vi "HVPSS_Single.vi"(0 "address":string="10.47.1.10", 1 "remote port or service name":u16=7, 4 "CONNECT":bool, 5 "SET":bool, 7 "FIFO_SIZE":u32=100, 9 "TRIG_DELAY":u32=50, 11 "TRIGGER_LEVEL":u32=10) -> (14 "Oscilloscope":waveform(dbl)(graph), 15 "DATA_AVAILABLE":bool, 18 "Timestamp":u64 format="%.0x", 19 "Halt":bool)   [LabVIEW 2019]
uses:
  Histogram/Histogram.lvlib
  <vilib>/Analysis/NI_AAL_SigProc.lvlib
  <vilib>/Analysis/NI_AALBase.lvlib
panel:
  in  "Tab Control":enum32{"ADC and Decimator", "pAmp CTRL"}(tab)
  in  "Full Scale Range":bool
  in  "DDR":bool
  in  "DCLK_RST":bool
  in  "ON":bool=TRUE
  in  "LED 1":bool
  in  "LED 0":bool=TRUE
  in  "CAL":bool
  in  "CAL_DLY":bool
  in  "OUTV":bool
  out "ADC500_CFG":u32=128
  in  "N":u32=1
  out "number":u32=9
  in  "SET POTS":bool
  in  "FINE OFFSET":u16(slide)=1023 scale=0.0..1023.0
  in  "OFFSET":u16(slide)=1023 scale=0.0..1024.0
  in  "HV_CTRL":bool
  out "RANGE 2":bool=TRUE
  out "RANGE 1":bool
  in  "RANGE":bool
  in  "LED":bool=TRUE
  in  "INIT":bool
  in  "Tab Control 2":T1(tab)
  in  "Trigger Edge":u32(ring)=3 items=["Falling Edge", "Rising Edge", "Auto", "EXT"]
  in  "CONTINOUS":bool
  in  "Counts":u32
  in  "GEN HISTO":bool
  in  "ENABLE":bool
  out "HISTOGRAM":u32[](graph)
  out "DONE":bool
  out "Progress":u32(slide) max=0
  out "STATUS":u32
  in  "Store Data":bool
  out "pAs_STATUS":u8[](array[numeric])=[1, 0, 0, 0, 9, 0, 0, 0]
  out "PAM_INIT_STATUS":u8[](array[numeric])
  out "ADC500_STATUS":u8[](array[numeric])
  out "DEC_STATUS":u8[](array[numeric])
  out "CONNECTED":bool
  out "BUSY":bool
  in  "Filename":path=path "/media/kbo/DATA/cernbox/DATA20211012/Cs137_dec2/Cs137_dec2.xlsx"
  out "output waveform":waveform(dbl)
  in  "threshold":dbl format="%0.2f"
  in  "width":i32=3 min=3
  in  "initialize (T)":bool=TRUE
  out "# found":i32
  out "Amplitudes":dbl[](array[numeric])
  in  "# bins":i32
  out "Histogram Graph":T2(graph)
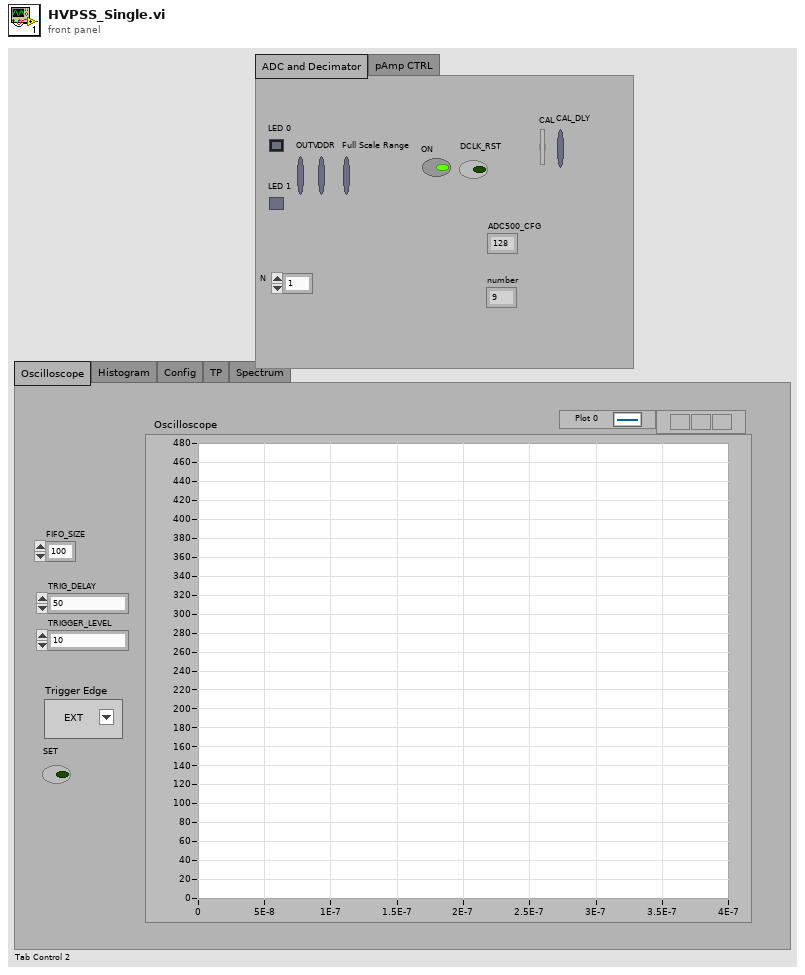
[diagram p1: front panel]
types:
  T1 = enum32{"Oscilloscope", "Histogram", "Config", "TP", "Spectrum"}
  T2 = cluster{"X Values":dbl[], "Histogram: h(x)":i32[]}
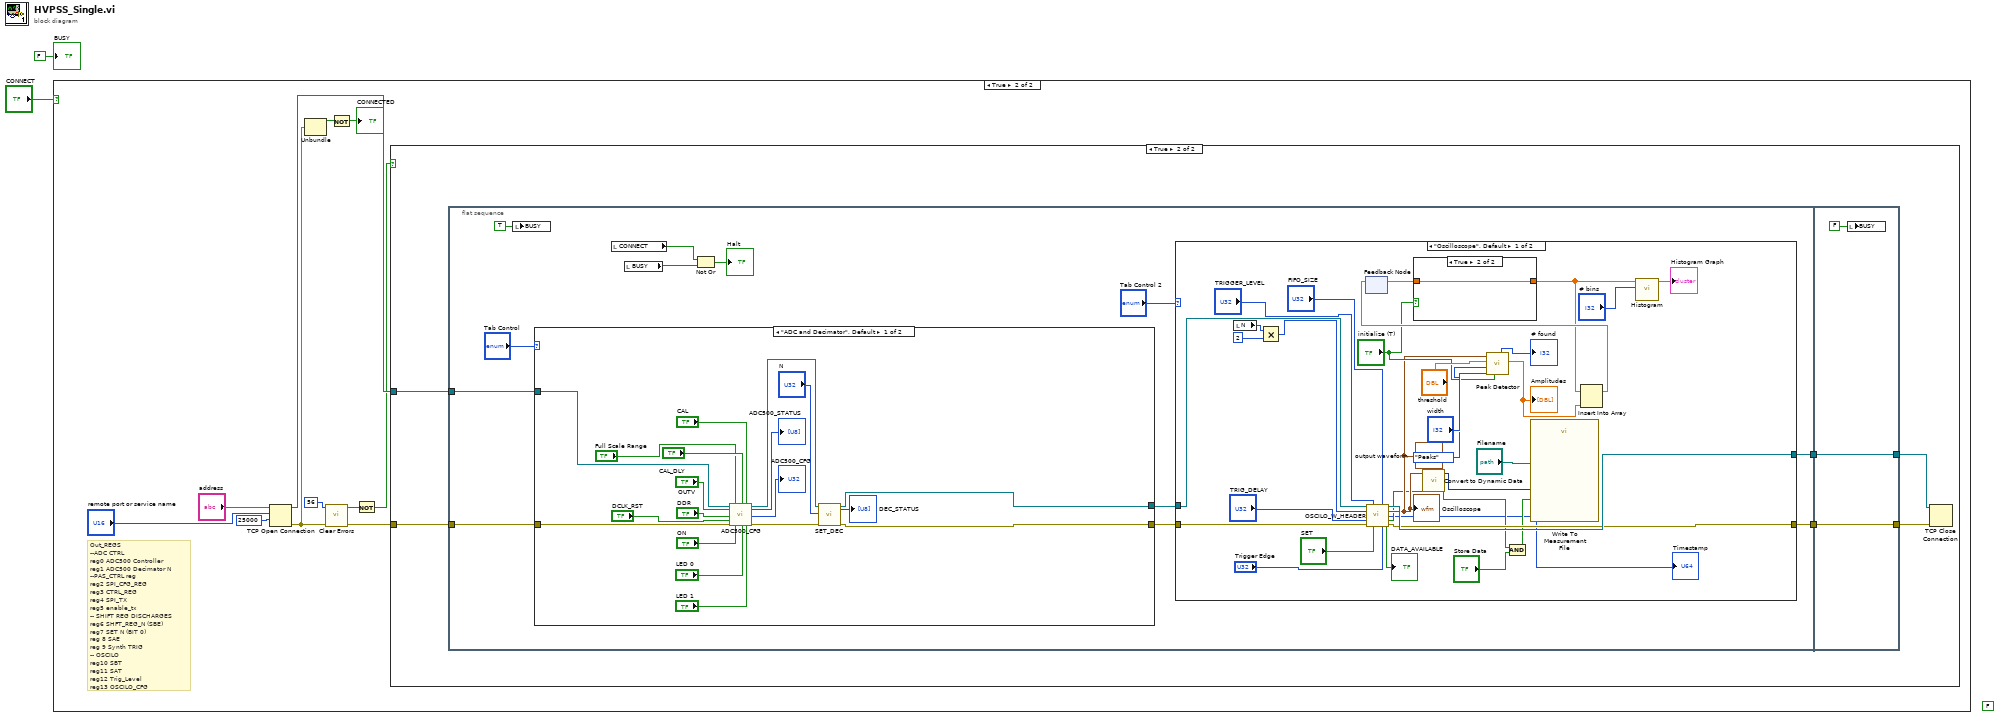
[diagram p0: block diagram]
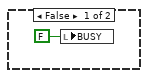
[diagram p3: hidden frame]
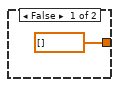
[diagram p4: hidden frame]
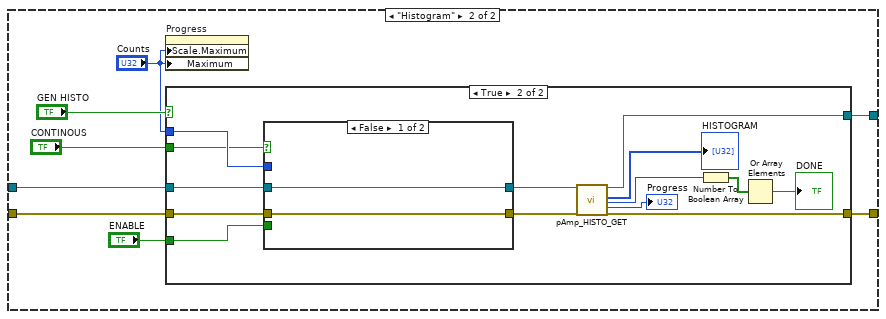
[diagram p5: hidden frame]
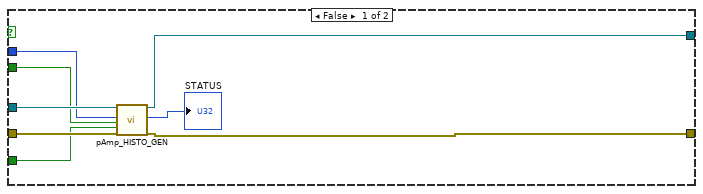
[diagram p6: hidden frame]
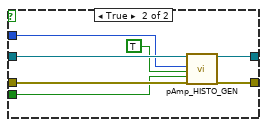
[diagram p7: hidden frame]
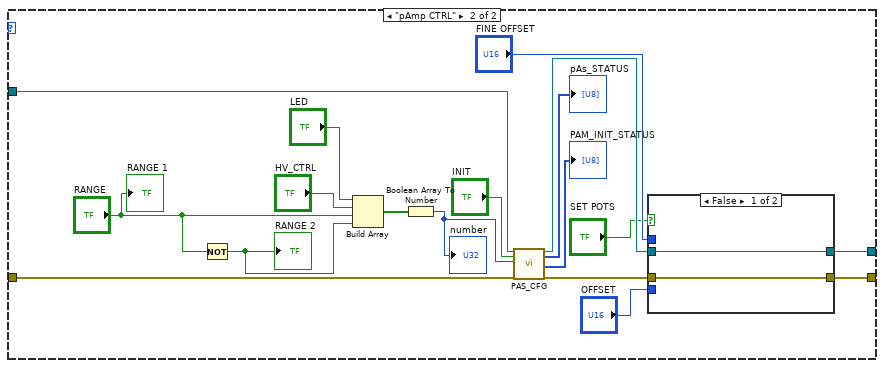
[diagram p8: hidden frame]
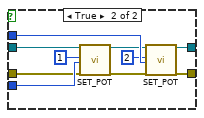
[diagram p9: hidden frame]
diagram:
  (unwired) FALSE
  n1 = case shown="True" "CONNECT" {
    frame False {
    }
    frame True {
      # "Out_REGS\n--ADC CTRL\nreg0 ADC500 Controller\nreg1 ADC500 Decimator N\n--PAS_CTRL reg\nreg2 SPI_CFG_REG\nreg3 CTRL_REG\nreg4 SPI_TX\nreg5 enable_tx\n-- SHIFT REG DISCHARGES\nreg6 SHFT_REG_N (SBE)\nreg7 SET N (BIT 0)\nreg 8 SAE\nreg 9 Synth TRIG\n-- OSCILO \nreg10 SBT\nreg11 SAT\nreg12 Trig_Level\nreg13 OSCILO_CFG"
      n2 = TCP Open Connection(address="address", remote port or service name="remote port or service name", timeout ms (60000)=25000) -> (connection ID=w13:refnum<k5>, error out=w7:errorcluster)  [unwired: 2 in]
      n3 = Unbundle(w7) -> ("status"=w12:bool)  [unwired: 2 out]
      n4 = call <vilib>:"Clear Errors.vi"("error in (no error)"=w7, "specific error code to clear (0: all)"=56) -> ("error out"=w5:errorcluster, "specific error cleared?"=w4:bool)  [unwired: 4 in]
      n5 = Not(x=w12) -> (.not. x?=→"CONNECTED":bool)
      n6 = Not(x=w4) -> (.not. x?=w3:bool)
      n7 = case shown="True" w3 {
        tunnel: w13 -> [_ w20]
        tunnel: w5 -> [_ w19]
        frame False {
          n8 = local write "BUSY"(FALSE ("BUSY")) -> ()
        }
        frame True {
          n9 = flat-sequence {
            tunnel: w20 -> [w32]
            tunnel: w19 -> [w31]
            tunnel: [w28] -> w16
            tunnel: [w27] -> w15
            tunnel: [w153] -> w18
            tunnel: [w155] -> w17
            tunnel: w16 -> [w155]
            tunnel: w15 -> [w153]
            frame #0 {
              n10 = local write "BUSY"(TRUE) -> ()
              n11 = case shown="\"ADC and Decimator\", Default" "Tab Control" {
                tunnel: [w106 w126] -> w29
                tunnel: [w104 w124] -> w25
                tunnel: w31 -> [w122 w134]
                tunnel: w32 -> [w121 w135]
                frame "ADC and Decimator", Default {
                  n12 = call "ADC500_CFG.vi"("TCP Network Connection in"=w121, "OUTV"="OUTV", "DDR"="DDR", "DCLK_RST"="DCLK_RST", "error in (no error)"=w122, "Full Scale Range"="Full Scale Range", "ON"="ON", "CAL_DLY"="CAL_DLY", "LED 0"="LED 0", "CAL"="CAL", "LED 1"="LED 1") -> ("TCP Network Connection out"=w109:refnum<k5>, "ADC500_STATUS"=→"ADC500_STATUS":u8[], "ADC500_CFG"=→"ADC500_CFG":u32, "error out"=w107:errorcluster)  [unwired: 5 in]
                  n13 = call "SET_DEC.vi"("TCP Network Connection in"=w109, "N"="N", "error in (no error)"=w107) -> ("TCP Network Connection out"=w106:refnum<k5>, "DEC_STATUS"=→"DEC_STATUS":u8[], "error out"=w104:errorcluster)  [unwired: 14 in]
                }
                frame "pAmp CTRL" {
                  n14 = Not(x="RANGE") -> (.not. x?=w137:bool)
                  "RANGE 2" <- w137
                  n15 = Build Array("LED", "HV_CTRL", "RANGE", w137) -> (w136:bool[])
                  n16 = Boolean Array To Number(Boolean array=w136) -> (number=w133:u32)
                  "number" <- w133
                  n17 = call "PAS_CFG.vi"("TCP Network Connection in"=w135, "INIT"="INIT", "pAs_REG"=w133, "error in (no error)"=w134) -> ("TCP Network Connection out"=w127:refnum<k5>, "pAs_STATUS"=→"pAs_STATUS":u8[], "PAM_INIT"=→"PAM_INIT_STATUS":u8[], "error out"=w125:errorcluster)  [unwired: 12 in]
                  n18 = case shown="False" "SET POTS" {
                    tunnel: "OFFSET" -> [_ w152]
                    tunnel: "FINE OFFSET" -> [_ w151]
                    tunnel: w127 -> [w142 w148]
                    tunnel: [w142 w146] -> w126
                    tunnel: w125 -> [w141 w145]
                    tunnel: [w141 w143] -> w124
                    frame False {
                    }
                    frame True {
                      n19 = call "SET_POT.vi"("TCP Network Connection in"=w148, "POT_N"=u32 1, "VALUE"=w152, "error in (no error)"=w145) -> ("TCP Network Connection out"=w147:refnum<k5>, "error out"=w144:errorcluster)  [unwired: 13 in, 1 out]
                      n20 = call "SET_POT.vi"("TCP Network Connection in"=w147, "POT_N"=u32 2, "VALUE"=w151, "error in (no error)"=w144) -> ("TCP Network Connection out"=w146:refnum<k5>, "error out"=w143:errorcluster)  [unwired: 13 in, 1 out]
                    }
                  }
                  "RANGE 1" <- "RANGE"
                }
              }
              n21 = local read "CONNECT"() -> (w23:bool)
              n22 = local read "BUSY"() -> (w22:bool)
              n23 = Not Or(1:w22, 2:w23) -> (0:→"Halt":bool)
              n24 = case shown="\"Oscilloscope\", Default" "Tab Control 2" {
                tunnel: w29 -> [w50 w72]
                tunnel: [w45 w70] -> w28
                tunnel: [w44 w69] -> w27
                tunnel: w25 -> [w48 w71]
                frame "Oscilloscope", Default {
                  n25 = local read "N"() -> (w41:u32)
                  n26 = Multiply(x=w41, y=u32 2) -> (x*y=w39:u32)
                  n27 = feedback #1() -> (w55:dbl[])  [unwired: 1 in]
                  n28 = call "OSCILO_W_HEADER.vi"("TCP Network Connection in"=w50, "TRIGGER_LEVEL"="TRIGGER_LEVEL", "FIFO_SIZE"="FIFO_SIZE", "dt (ns)"=w39, "TRIG_DELAY"="TRIG_DELAY", "error in (no error)"=w48, "SET"="SET", "Trigger Edge"="Trigger Edge") -> ("TCP Network Connection out"=w45:refnum<k5>, "output waveform"=w38:waveform(dbl), "Timestamp"=→"Timestamp":u64, "DATA_AVAILABLE"=w37:bool, "error out"=w44:errorcluster)  [unwired: 3 in]
                  "Oscilloscope" <- w38
                  "output waveform" <- w38
                  "DATA_AVAILABLE" <- w37
                  n29 = case shown="True" "initialize (T)" {
                    tunnel: [dbl[] [] w64] -> w51
                    tunnel: w55 -> [_ w64]
                    frame False {
                    }
                    frame True {
                    }
                  }
                  n30 = call "Convert to Dynamic Data"("Array"=w38) -> ("Dynamic Data Type"=w52:dynamicdata)  [unwired: 3 in]
                  n31 = call <vilib>:"Peak Detector.vi"("initialize (T)"="initialize (T)", "peaks/valleys"=enum32{"Peaks", "Valleys"}."Peaks", "width"="width", "threshold"="threshold", "X"=w38) -> ("Amplitudes"=w57:dbl[], "# found"=→"# found":i32)  [unwired: 2 in, 3 out]
                  "Amplitudes" <- w57
                  n32 = And(x=w37, y="Store Data") -> (x .and. y?=w36:bool)
                  n33 = call "Write To Measurement File"("Signals"=w52, "Enable"=w36, "Filename"="Filename") -> ()  [unwired: 14 in, 3 out]
                  n34 = Insert Into Array(array=w51, new element=w57) -> (w56:dbl[])  [unwired: 1 in]
                  n35 = feedback-in #1(w56) -> ()
                  n36 = call <vilib>:"Histogram.vi"("intervals"="# bins", "X"=w51) -> ("Histogram Graph"=→"Histogram Graph":T2)  [unwired: 6 in, 3 out]
                }
                frame "Histogram" {
                  n37 = property on="Progress" class="Slide (strict)"("Scale.Maximum"="Counts", "Maximum"="Counts") -> ()  [unwired: 2 in, 2 out]
                  n38 = case shown="True" "GEN HISTO" {
                    tunnel: w72 -> [w80 w84]
                    tunnel: w71 -> [w79 w85]
                    tunnel: [w74 w89] -> w70
                    tunnel: [w73 w88] -> w69
                    tunnel: "ENABLE" -> [w75 w81]
                    tunnel: "Counts" -> [w78 w83]
                    tunnel: "CONTINOUS" -> [w77 w82]
                    frame False {
                      n39 = call "pAmp_HISTO_GEN.vi"("TCP Network Connection in"=w80, "COUNTS"=w78, "CONTINOUS"=w77, "ENABLE"=w75, "error in (no error)"=w79) -> ("TCP Network Connection out"=w74:refnum<k5>, "STATUS"=→"STATUS":u32, "error out"=w73:errorcluster)  [unwired: 12 in]
                    }
                    frame True {
                      n40 = case shown="False" w82 {
                        tunnel: [w96 w103] -> w87
                        tunnel: [w95 w102] -> w86
                        tunnel: w85 -> [w95 w100]
                        tunnel: w84 -> [w96 w101]
                        tunnel: w83 -> [_ w99]
                        tunnel: w81 -> [_ w97]
                        frame False {
                        }
                        frame True {
                          n41 = call "pAmp_HISTO_GEN.vi"("TCP Network Connection in"=w101, "COUNTS"=w99, "CONTINOUS"=TRUE, "ENABLE"=w97, "error in (no error)"=w100) -> ("TCP Network Connection out"=w103:refnum<k5>, "error out"=w102:errorcluster)  [unwired: 12 in, 1 out]
                        }
                      }
                      n42 = call "pAmp_HISTO_GET.vi"("TCP Network Connection in"=w87, "error in (no error)"=w86) -> ("TCP Network Connection out"=w89:refnum<k5>, "Oscilloscope"=→"HISTOGRAM":u32[], "DONE"=w92:u32, "CURR_COUNT"=→"Progress":u32, "error out"=w88:errorcluster)  [unwired: 12 in, 1 out]
                      n43 = Number To Boolean Array(number=w92) -> (Boolean array=w91:bool[])
                      n44 = Or Array Elements(Boolean array=w91) -> (logical OR=→"DONE":bool)
                    }
                  }
                }
              }
            }
            frame #1 {
              n45 = local write "BUSY"(FALSE) -> ()
            }
          }
          n46 = TCP Close Connection(connection ID=w17, error in (no error)=w18) -> ()  [unwired: 1 in, 2 out]
        }
      }
    }
  }
  "BUSY" <- FALSE ("BUSY")
